vi "ctrl ui.vi"() -> ()   [LabVIEW 2013, in "control label adjustment.lvclass"]
uses:
  control label adjustment.lvclass
  <vilib>/CEF_TreeControl/Node/NodeRef.ctl
  <vilib>/CEF_TreeControl/Node/NISE_CEF_Node.lvclass
  <vilib>/NI/AMC/Message Queue.ctl
  <vilib>/NI/AMC/Message.ctl
  <vilib>/NI/Tools/Keyed Array/KeyedArray.ctl
  <vilib>/CEF_TreeControl/Node/UserEventRef.ctl
  <vilib>/CEF_TreeControl/Controls/EventCluster.ctl
  control label adjustment.lvclass/control label adjustment.ctl
  Read font name (App Font).vi
  Read font size (15).vi
  Read make lower case (F).vi
  Read set font (F).vi
  <vilib>/NI/Tools/Keyed Array/Tools_KeyedArray.lvlib
  <vilib>/NI/AMC/AMC.lvlib
  <vilib>/CEF_TreeControl/NISE_CEF_TreeControl.lvlib
panel:
  in  "user event":T1
  in  "main queue":T2
  in  "node ref":T3
  in  "font name (App Font)":string="App Font"
  in  "font size (15)":u32=15
  in  "make lower case (F)":bool
  in  "set font (F)":bool
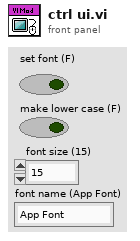
[diagram p1: front panel]
types:
  T1 = typedef "NISE_CEF_Node.lvclass/UserEventRef.ctl" = refnum<user-event>
  T2 = typedef "AMC.lvlib/Message Queue.ctl" = refnum<queue>
  T3 = typedef "NISE_CEF_Node.lvclass/NodeRef.ctl" = refnum<data-value>
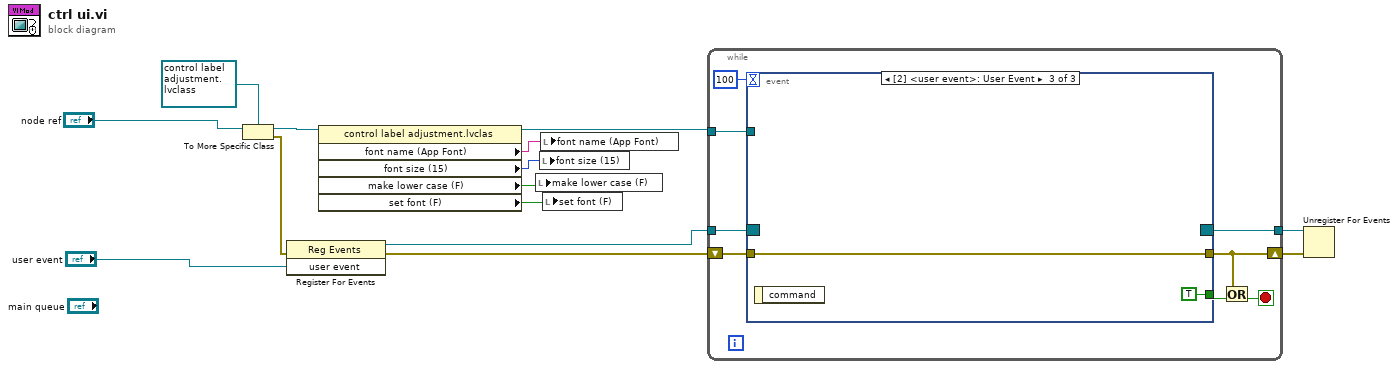
[diagram p0: block diagram]
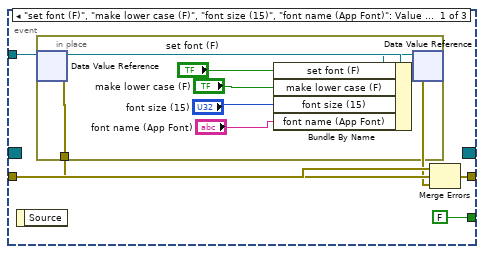
[diagram p2: hidden frame]
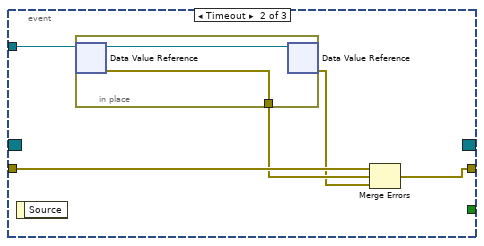
[diagram p3: hidden frame]
diagram:
  n1 = To More Specific Class(target class=refnum<data-value> refnum, reference="node ref") -> (specific class reference=w10:refnum<data-value>, error out=w9:errorcluster)  [unwired: 1 in]
  n2 = register-events(error in=w9, "user event") -> (reference out=w13:refnum<event-registration>, error out=w14:errorcluster)  [unwired: 1 in]
  n3 = property class="control label adjustment.lvclas"(reference=w10) -> (reference out=w7:refnum<data-value>, "font name (App Font)"=w3:string, "font size (15)"=w4:u32, "make lower case (F)"=w6:bool, "set font (F)"=w5:bool)  [unwired: 1 in, 1 out]
  n4 = local write "make lower case (F)"(w6) -> ()
  n5 = local write "font size (15)"(w4) -> ()
  n6 = local write "font name (App Font)"(w3) -> ()
  n7 = local write "set font (F)"(w5) -> ()
  n8 = while {
    shift-right: [w15] -> w12
    shift-left: w14 -> [w19]
    tunnel: w13 -> [w22]
    tunnel: [w21] -> w11
    tunnel: w7 -> [w18]
    stop <- w16 stop-if-true
    n9 = event shown="[2] <user event>: User Event" {
      selector: w22 -> [_ _ _]
      dyn-events: [_ _ _] -> w21
      timeout: 100 -> [_ _ _]
      tunnel: [FALSE _ TRUE] -> w20
      tunnel: [w26 w38 w44] -> w15
      tunnel: w19 -> [w28 w39 w44]
      tunnel: w18 -> [w27 w40 _]
      event "set font (F)", "make lower case (F)", "font size (15)", "font name (App Font)": Value Change {
        n10 = event-data() -> ()  [unwired: 1 in, 1 out]
        n11 = in-place {
          in-place-border: [w33] -> w24
          n12 = in-place-dvr #1(w27) -> (w35:refnum<class "control label adjustment.lvclass">, w33:errorcluster)
          n13 = Bundle By Name(cluster=w35, "set font (F)"="set font (F)", "make lower case (F)"="make lower case (F)", "font size (15)"="font size (15)", "font name (App Font)"="font name (App Font)") -> (w34:refnum<class "control label adjustment.lvclass">)
          n14 = in-place-dvr #1(w34) -> (w23:errorcluster)  [unwired: 1 out]
        }
        n15 = Merge Errors(w28, w24, w23) -> (w26:errorcluster)
      }
      event Timeout {
        n16 = event-data() -> ()  [unwired: 1 in, 1 out]
        n17 = in-place {
          in-place-border: [w41] -> w37
          n18 = in-place-dvr #2(w40) -> (w42:refnum<class "control label adjustment.lvclass">, w41:errorcluster)
          n19 = in-place-dvr #2(w42) -> (w36:errorcluster)  [unwired: 1 out]
        }
        n20 = Merge Errors(w39, w37, w36) -> (w38:errorcluster)
      }
      event User Event {
        n21 = event-data() -> ()  [unwired: 1 in, 1 out]
      }
    }
    n22 = Or(x=w15, y=w20) -> (x .or. y?=w16:bool)
  }
  n23 = Unregister For Events(event registration refnum=w11, error in=w12) -> ()  [unwired: 1 out]
